vi "Write Data.vi"(8 "error in (no error)":errorcluster, 10 "Data":string, 11 "StringStream in":refnum<class "StringStream.lvclass">) -> (0 "error out":errorcluster, 3 "StringStream out":refnum<class "StringStream.lvclass">)   [LabVIEW 2020, in "IO.lvlib" / "StringStream.lvclass"]
uses:
  StringStream.lvclass
  StringStream.lvclass/StringStream.ctl
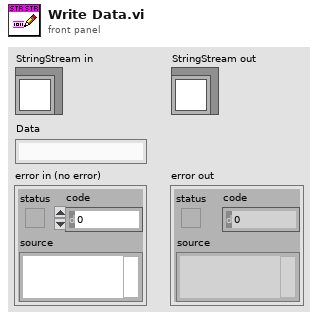
[diagram p1: front panel]
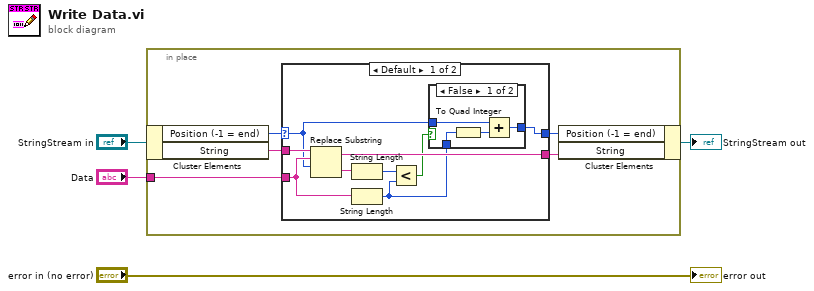
[diagram p0: block diagram]
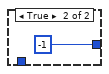
[diagram p2: hidden frame]
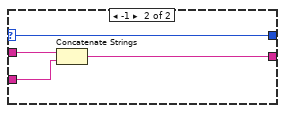
[diagram p3: hidden frame]
diagram:
  n1 = in-place "In Place Element Structure" {
    in-place-border: "Data" -> [w8]
    n2 = in-place-cluster #1("StringStream in") -> ("Position (-1 = end)"=w6:i64, "String"=w9:string)
    n3 = case shown="Default" w6 {
      selector: w6 -> [w12 w24]
      tunnel: w9 -> [w18 w27]
      tunnel: w8 -> [w17 w26]
      tunnel: [w16 w25] -> w7
      tunnel: [w11 w24] -> w5
      frame Default {
        n4 = Replace Substring(3:w12, 4:w17, 5:w18) -> (0:w15:string, 1:w16:string)  [unwired: 1 in]
        n5 = String Length(string=w15) -> (length=w14:i32)
        n6 = String Length(string=w17) -> (length=w10:i32)
        n7 = Less?(x=w14, y=w10) -> (x < y?=w13:bool)
        n8 = case shown="False" w13 {
          tunnel: w12 -> [w21 _]
          tunnel: [w19 i64 -1 ("Position (-1 = end)")] -> w11
          tunnel: w10 -> [w22 _]
          frame False {
            n9 = To Quad Integer(1:w22) -> (0:w20:i64)
            n10 = Add(x=w21, y=w20) -> (x+y=w19:i64)
          }
          frame True {
          }
        }
      }
      frame -1 {
        n11 = Concatenate Strings(w27, w26) -> (w25:string)
      }
    }
    n12 = in-place-cluster #1("Position (-1 = end)"=w5, "String"=w7) -> (→"StringStream out":refnum<class "StringStream.lvclass">)
  }
  "error out" <- "error in (no error)"
